vi "Set Rate (RPM).vi"(8 "error in (no error)":errorcluster, 10 "Rate (RPM)":dbl, 11 "Motors with Encoders in":refnum<class "Motors with Encoders.lvclass">) -> (0 "error out":errorcluster, 3 "Motors with Encoders out":refnum<class "Motors with Encoders.lvclass">)   [LabVIEW 2014, in "Motors with Encoders.lvlib" / "Motors with Encoders.lvclass"]
uses:
  Motors with Encoders.lvclass
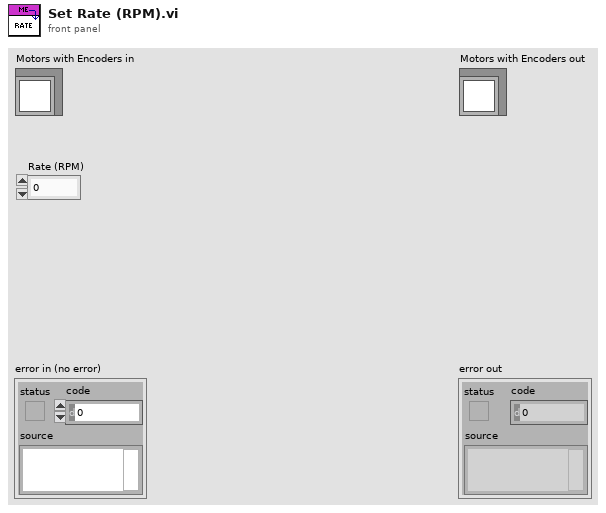
[diagram p1: front panel]
types:
  T1 = typedef "Motors with Encoders.lvlib/Motors with Encoders.lvclass/Motors with Encoders State.ctl" = cluster{"Forward Switch":bool, "Reverse Switch":bool, "Measured RPM":dbl, "Distance (in)":dbl, "Setpoint RPM":dbl, "Encoder Count":i64, "Home Count":i64, "Config":T2}
  T2 = typedef "Motors with Encoders.lvlib/Motors with Encoders.lvclass/Motors with Encoders Config.ctl" = cluster{"Counts  Per Revolution":u32, "Invert Encoder Direction":bool, "Diameter of Revolution":dbl, "Max RPM":dbl, "Encoder Control":bool}
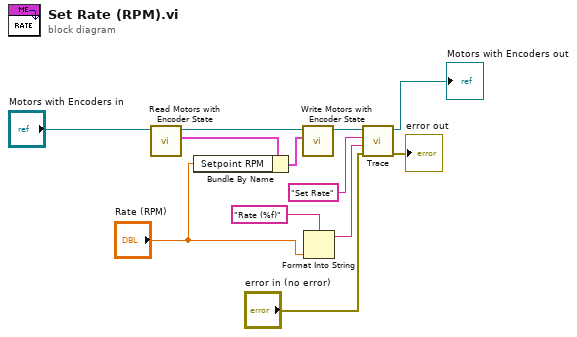
[diagram p0: block diagram]
diagram:
  n1 = call-dynamic "Read Motors with Encoder State.vi"("Motors with Encoders in"="Motors with Encoders in") -> ("Motors with Encoder State"=w4:T1, "Motors with Encoders out"=w5:refnum<class "Motors with Encoders.lvclass">)  [unwired: 8 in, 1 out]
  n2 = Bundle By Name(cluster=w4, "Setpoint RPM"="Rate (RPM)") -> (w3:T1)
  n3 = call-dynamic "Write Motors with Encoder State.vi"("Motors with Encoder State"=w3, "Motors with Encoders in"=w5) -> ("Motors with Encoders out"=w1:refnum<class "Motors with Encoders.lvclass">)  [unwired: 8 in, 1 out]
  n4 = Format Into String(format string="Rate (%f)", "Rate (RPM)") -> (resulting string=w7:string)  [unwired: 2 in, 1 out]
  n5 = call-dynamic "Trace.vi"("error in (no error)"="error in (no error)", "System Message"=w7, "System Action"="Set Rate", "System Actor in"=w1) -> ("error out"=→"error out":errorcluster, "System Actor out"=→"Motors with Encoders out":refnum<class "Motors with Encoders.lvclass">)  [unwired: 6 in]
